vi "Write RunVirtual.vi"(8 "error in (no error)":errorcluster, 10 "RunVirtual":bool, 11 "DriveTrain in":refnum<class "DriveTrain.lvclass">) -> (0 "error out":errorcluster, 3 "DriveTrain out":refnum<class "DriveTrain.lvclass">)   [LabVIEW 2013, in "DriveTrain.lvlib" / "DriveTrain.lvclass"]
uses:
  DriveTrain.lvclass
  DriveTrain.lvclass/DriveTrain.ctl
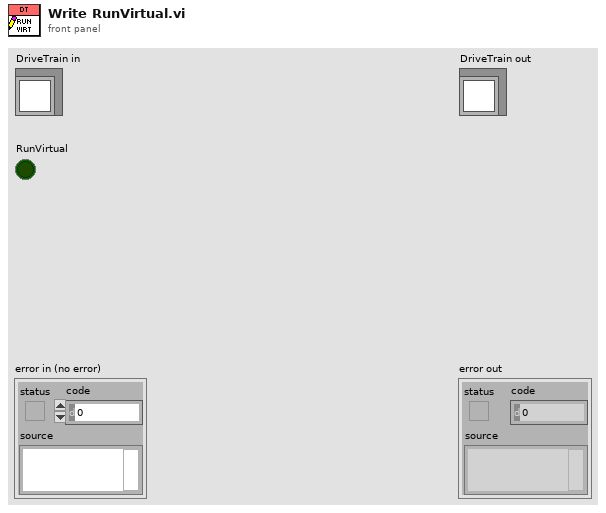
[diagram p1: front panel]
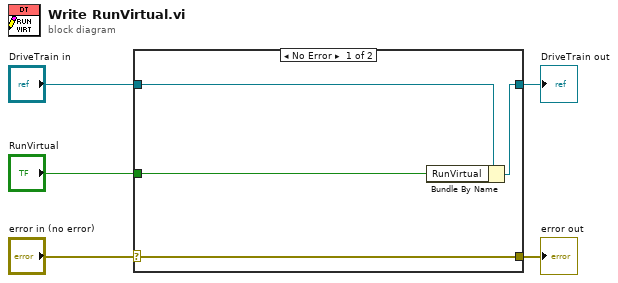
[diagram p0: block diagram]
diagram:
  n1 = case shown="No Error" "error in (no error)" {
    selector: "error in (no error)" -> [w9 w10]
    tunnel: [w9 w10] -> w4
    tunnel: [w7 w11] -> w2
    tunnel: "DriveTrain in" -> [w8 w11]
    tunnel: "RunVirtual" -> [w6 _]
    frame No Error {
      n2 = Bundle By Name(cluster=w8, "RunVirtual"=w6) -> (w7:refnum<class "DriveTrain.lvclass">)
    }
    frame Error {
    }
  }
  "error out" <- w4
  "DriveTrain out" <- w2
